vi "Intake Immediate Wrapper.vi"() -> ()   [LabVIEW 2019]
uses:
  Implementation/Intake Operations.ctl
panel:
  in  "Intake Power":dbl
  in  "Operation":T1
  in  "Pivot Position":dbl
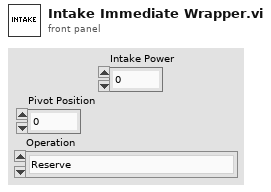
[diagram p1: front panel]
types:
  T1 = typedef "Intake Operations.ctl" = enum16{"Reserve", "Read Current", "Immediate Setpoints", "Pivot Down"}
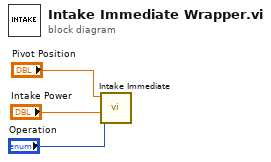
[diagram p0: block diagram]
diagram:
  n1 = call "Intake Immediate.vi"("Operation"="Operation", "Intake Power"="Intake Power", "Pivot Position"="Pivot Position") -> ()  [unwired: 8 in, 1 out]
